vi "CreateBankNode.vi"(7 "DOM Document":refnum<k20>, 8 "Error In":errorcluster, 11 "Bank Configuration":T1) -> (0 "Error Out":errorcluster, 3 "Bank Channel Node":refnum<k20>)   [LabVIEW 2012]
uses:
  BankConfiguration.ctl
  libs/LV-Utilities/LV-Utilities.lvlib
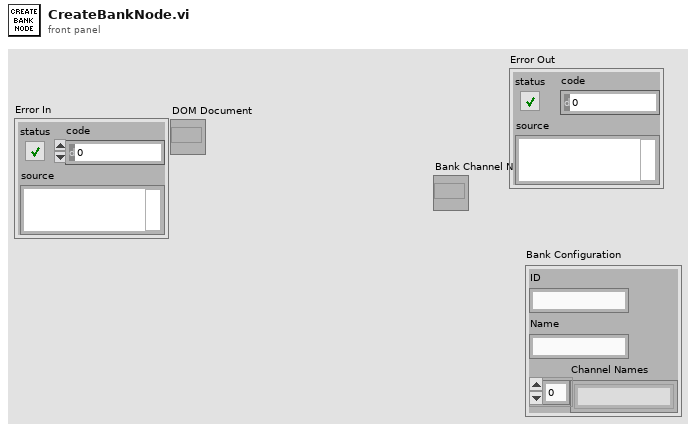
[diagram p1: front panel]
types:
  T1 = typedef "BankConfiguration.ctl" = cluster{"ID":string, "Name":string, "Channel Names":string[]}
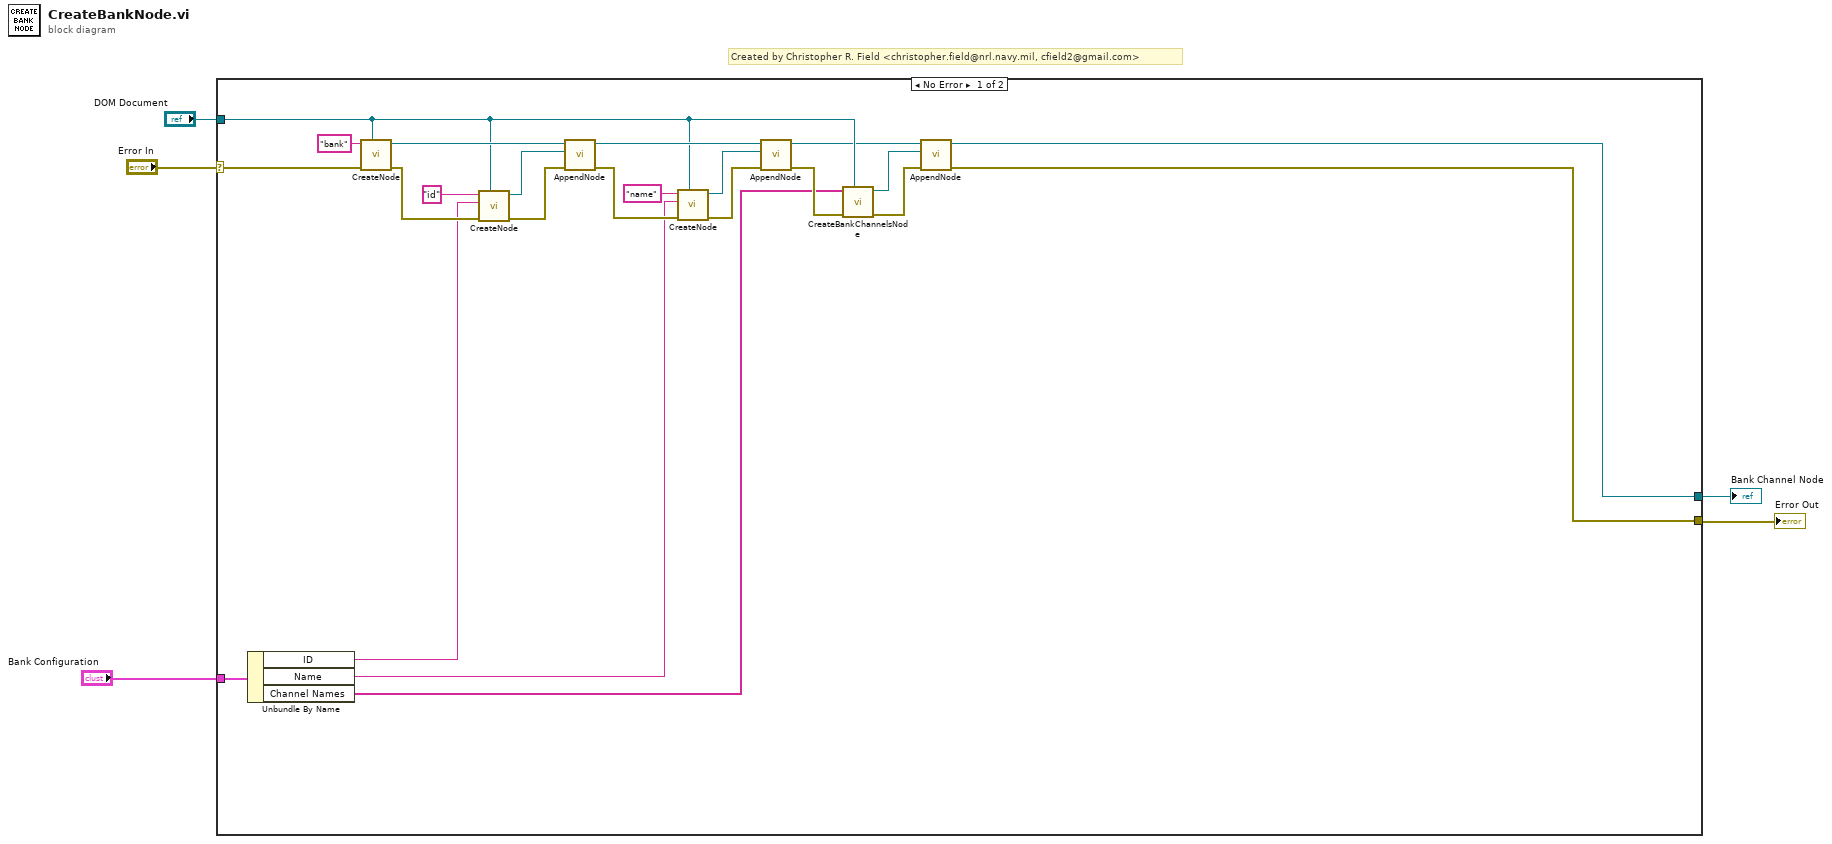
[diagram p0: block diagram]
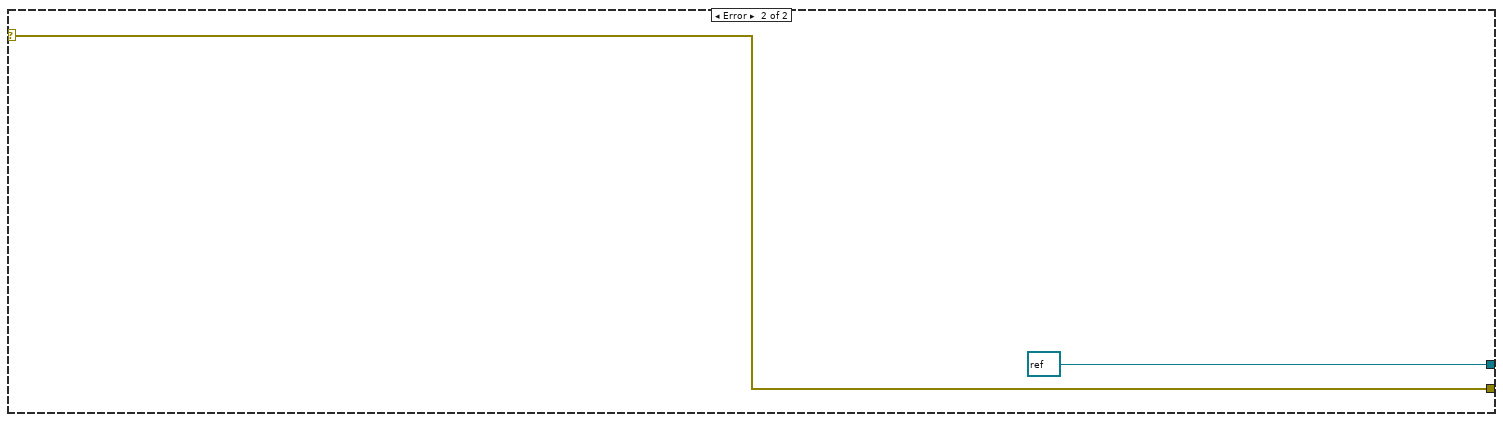
[diagram p2: hidden frame]
diagram:
  # "Created by Christopher R. Field <christopher.field@nrl.navy.mil, cfield2@gmail.com>"
  n1 = case shown="No Error" "Error In" {
    selector: "Error In" -> [w28 w30]
    tunnel: "DOM Document" -> [w13 _]
    tunnel: [w6 w30] -> w3
    tunnel: [w7 refnum<k20> refnum ("Wirings Node 2")] -> w2
    tunnel: "Bank Configuration" -> [w25 _]
    frame No Error {
      n2 = Unbundle By Name(w25) -> ("ID"=w23:string, "Name"=w17:string, "Channel Names"=w11:string[])
      n3 = call "CreateNode.vi"("DOM Document"=w13, "Error In"=w28, "Tag Name"="bank") -> ("Error out"=w26:errorcluster, "Node"=w22:refnum<k20>)  [unwired: 7 in]
      n4 = call "CreateNode.vi"("DOM Document"=w13, "Error In"=w26, "Text"=w23, "Tag Name"="id") -> ("Error out"=w20:errorcluster, "Node"=w21:refnum<k20>)  [unwired: 6 in]
      n5 = call "AppendNode.vi"("Error In"=w20, "Child Node"=w21, "Parent Node In"=w22) -> ("Error Out"=w19:errorcluster, "Parent Node Out"=w16:refnum<k20>)  [unwired: 7 in]
      n6 = call "CreateNode.vi"("DOM Document"=w13, "Error In"=w19, "Text"=w17, "Tag Name"="name") -> ("Error out"=w14:errorcluster, "Node"=w15:refnum<k20>)  [unwired: 6 in]
      n7 = call "AppendNode.vi"("Error In"=w14, "Child Node"=w15, "Parent Node In"=w16) -> ("Error Out"=w12:errorcluster, "Parent Node Out"=w10:refnum<k20>)  [unwired: 7 in]
      n8 = call "CreateBankChannelsNode.vi"("DOM Document"=w13, "Error In"=w12, "Channel Names"=w11) -> ("Error Out"=w9:errorcluster, "Channel Node"=w8:refnum<k20>)  [unwired: 7 in]
      n9 = call "AppendNode.vi"("Error In"=w9, "Child Node"=w8, "Parent Node In"=w10) -> ("Error Out"=w6:errorcluster, "Parent Node Out"=w7:refnum<k20>)  [unwired: 7 in]
    }
    frame Error {
    }
  }
  "Bank Channel Node" <- w2
  "Error Out" <- w3
